vi "SV Append Data (1 Ch) ([DBL]).vi"(7 "reset (F)":bool, 10 "maximum length (-1 = unlimited)":i32=-1, 11 "data in":dbl[](array[numeric])) -> (3 "appended data":dbl[](array[numeric]))   [LabVIEW 2017]
doc: "Use this VI to buffer data by appending input data to previously buffered data. Set the <B>maximum length</B> to set the buffered array size. The VI functions like a FIFO (First In, First Out) buffer, meaning that the oldest data is overwritten as new elements are added to the buffer. Wire data to the <B>data in</B> input to determine the polymorphic instance to use or manually select the instance."
uses:
  <vilib>/addons/_NISVFA/_Shared subVIs/Common/svc_Get Array Subset (Index).vi
  <vilib>/addons/_NISVFA/_Shared subVIs/Common/svc_Coerce Index and Length.vi
  <vilib>/addons/_NISVFA/_Shared subVIs/Common/svc_Conditional Merge Error.vi
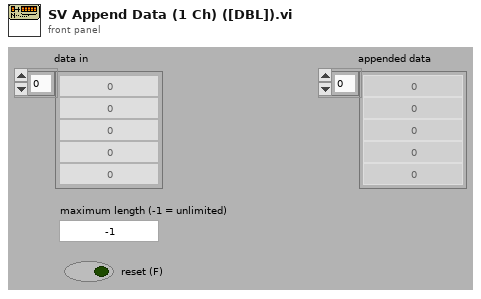
[diagram p1: front panel]
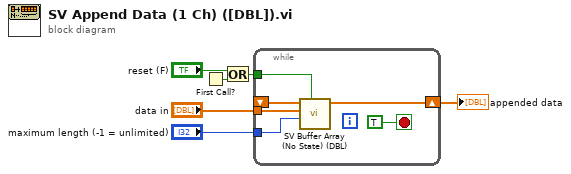
[diagram p0: block diagram]
diagram:
  n1 = First Call?() -> (First Call?: T/F=w1:bool)
  n2 = Or(x="reset (F)", y=w1) -> (x .or. y?=w5:bool)
  n3 = while {
    tunnel: "data in" -> [w7]
    shift-right: [w12] -> w4
    shift-left: _ -> [w11]
    tunnel: "maximum length (-1 = unlimited)" -> [w8]
    tunnel: w5 -> [w10]
    stop <- TRUE stop-if-true
    n4 = call <vilib>:"SV Buffer Array (No State) (DBL).vi"("clear buffer (False)"=w10, "buffer length  [samples] (-1 = unlimited)"=w8, "Y"=w7, "buffer in"=w11) -> ("buffer out"=w12:dbl[])  [unwired: 7 in]
  }
  "appended data" <- w4
